vi "example_vi_1.vi"() -> ()   [LabVIEW 2015]
panel:
  out "new boolean":bool
  out "new string":string
  out "new number":dbl
  out "array element":u8
  out "new array":u8[](array[slide]) scale=0.0..100.0
  in  "starting string":string
  in  "starting boolean":bool
  in  "starting number":dbl
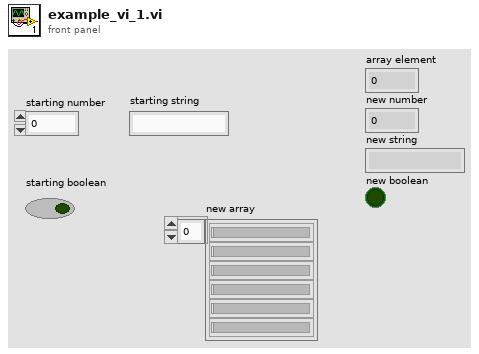
[diagram p1: front panel]
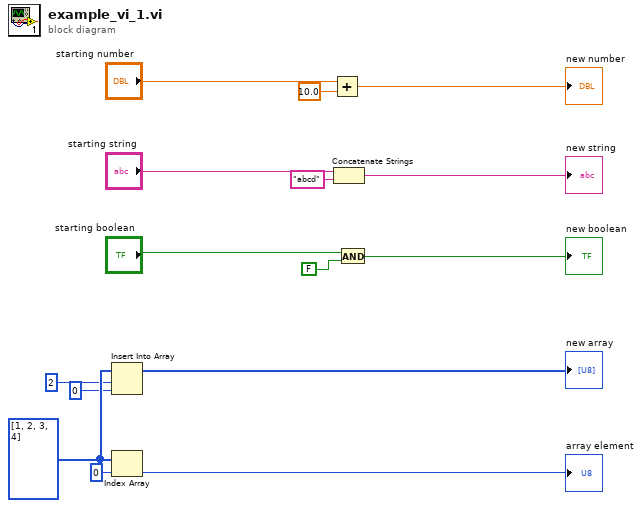
[diagram p0: block diagram]
diagram:
  w11 = u8[] [1, 2, 3, 4]
  n1 = Insert Into Array(array=w11, index=2, new element=0 ("new element/subarray")) -> (→"new array":u8[])
  n2 = Index Array(array=w11, index=0) -> (element=→"array element":u8)
  n3 = Add(x="starting number", y=10.0) -> (x+y=→"new number":dbl)
  n4 = Concatenate Strings("starting string", "abcd" ("string")) -> (→"new string":string)
  n5 = And(x="starting boolean", y=FALSE) -> (x .and. y?=→"new boolean":bool)
